vi "RT_Control_Adrian_AllIncluded_NoAngles.vi"(10 "rt fifo":refnum<k33>, 11 "Parameters":T1) -> (0 "error out":errorcluster, 2 "Delayed Cycles":dbl)   [LabVIEW 2021]
uses:
  parametersRT.ctl
  <vilib>/DAQmx/write.llb/DAQmx Write (Analog 1D DBL NChan 1Samp).vi
  <vilib>/DAQmx/read.llb/DAQmx Read (Analog 1D DBL NChan 1Samp).vi
  <vilib>/DAQmx/configure/timing.llb/DAQmx Timing (Sample Clock).vi
  <vilib>/DAQmx/miscellaneous.llb/DAQmx Fill In Error Info.vi
  <resource>/objmgr/daqmx.rc
panel:
  out "error out 7":errorcluster
  out "error out 6":errorcluster
  out "error out 5":errorcluster
  out "error out 4":errorcluster
  out "error out 2":errorcluster
  out "FB Raw Readings":dbl[][](array[numeric])
  in  "Stop Loop":bool
  in  "System Information":enum32{"RT System"}(tab)
  in  "source":tag
  in  "source 2":tag
  in  "RT Data Monitoring":enum32{"Forces", "Angles", "Power", "Pressure"}(tab)
  out "Bias Voltages":dbl[][](array[numeric])=[[-0.0710179470114859, -0.17463349299050945, -0.11016159714741332, 0.026018829634351103, 0.12897648926553976, 0.08259620236774425]]
  out "Bias Vector":dbl[](array[numeric])=[-0.0710179470114859, -0.17463349299050945, -0.11016159714741332, 0.026018829634351103, 0.12897648926553976, 0.08259620236774425]
  in  "Bias":bool
  in  "Unbias":bool
  # "Important! Set angle offset before reading angles"
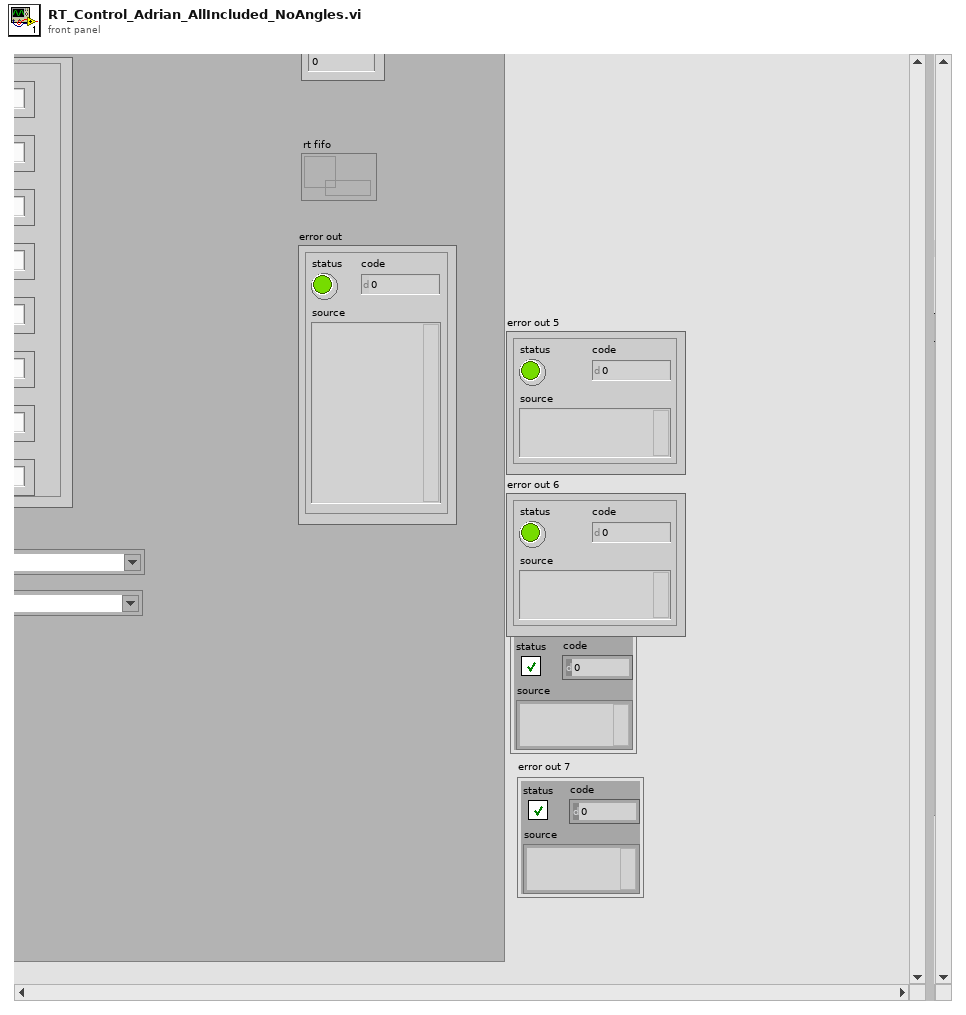
[diagram p1: front panel]
types:
  T1 = typedef "parametersRT.ctl" = cluster{"N_Signals_FIFO":u32, "Input Rate (Hz)":dbl, "Acq Time (s)":dbl, "NumOfWarmupIters":u32, "Size fifo":u32, "Period NCL (ms)":i64, "Timeout fifo Read":i32, "Size Sent Array":i32}
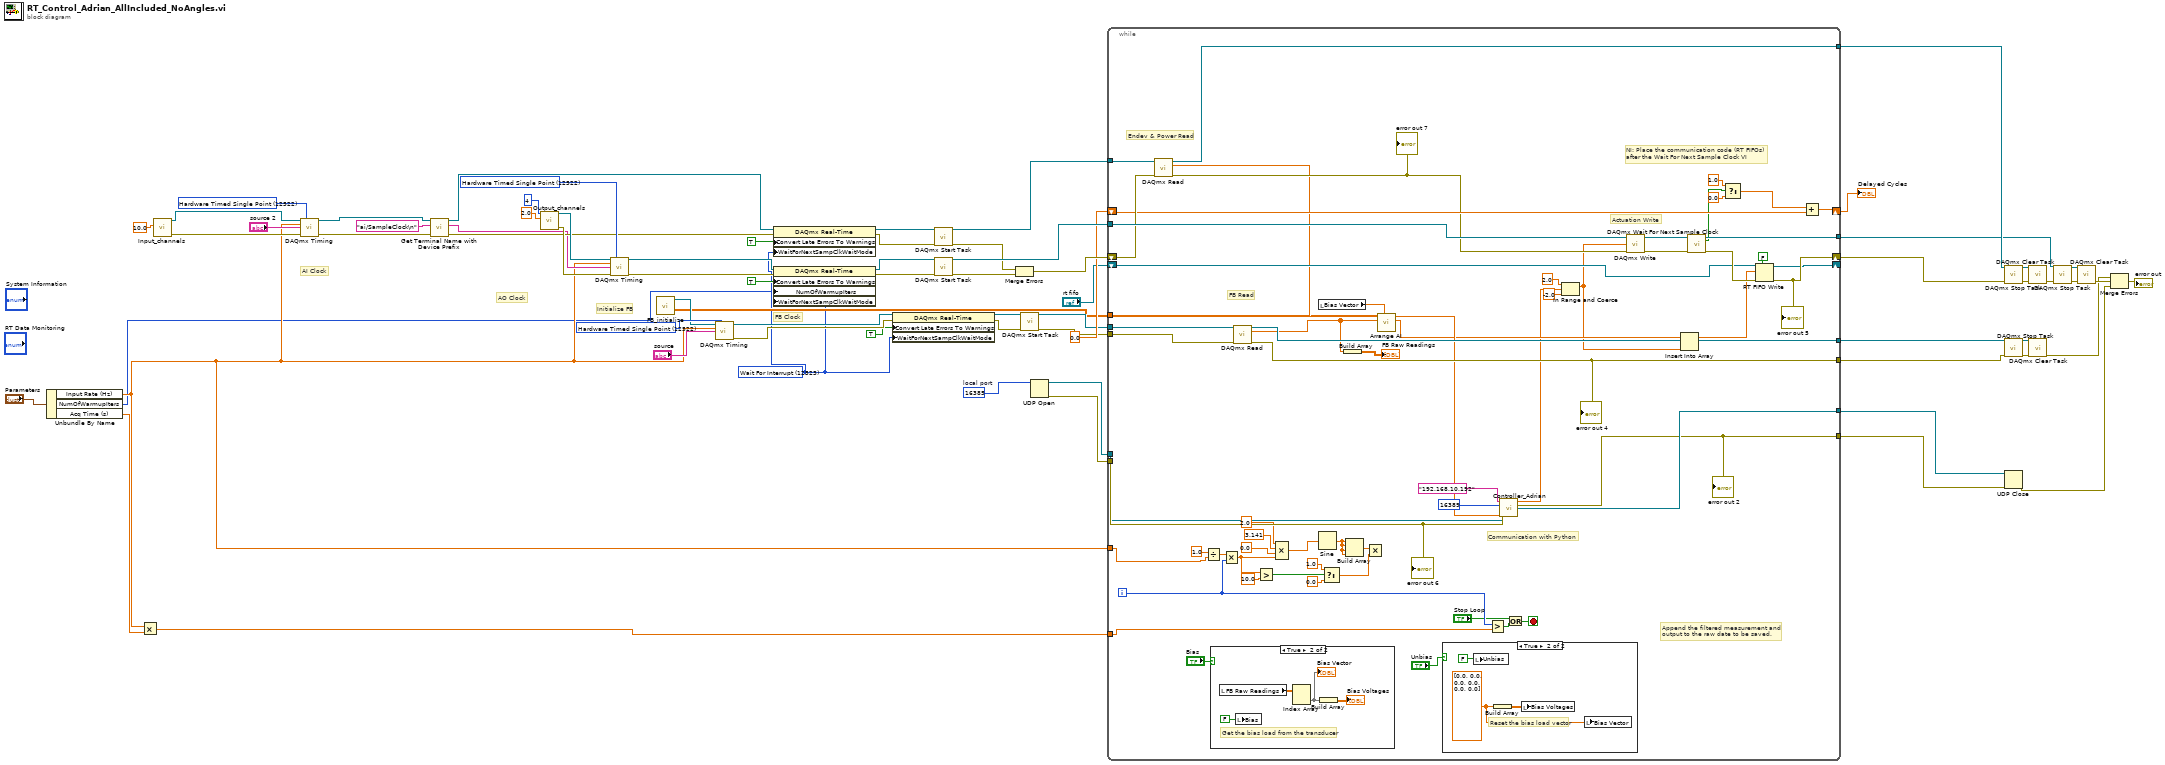
[diagram p0: block diagram]
diagram:
  w2 = 12523 items=["Wait For Interrupt"=12523, "Poll"=12524, "Yield"=12525] ("WaitForNextSampClkWaitMode")
  w34 = 12522 items=["Finite Samples"=10178, "Continuous Samples"=10123, "Hardware Timed Single Point"=12522] ("sample mode")
  w44 = u16 16385  # local port
  w51 = 12522 items=["Finite Samples"=10178, "Continuous Samples"=10123, "Hardware Timed Single Point"=12522] ("sample mode")
  w69 = 12522 items=["Finite Samples"=10178, "Continuous Samples"=10123, "Hardware Timed Single Point"=12522] ("sample mode")
  # "Initialize FB"
  # "AO Clock"
  # "AI Clock"
  # "FB Clock"
  n1 = Unbundle By Name("Parameters") -> ("Input Rate (Hz)"=w3:dbl, "NumOfWarmupIters"=w1:u32, "Acq Time (s)"=w64:dbl)
  n2 = Multiply(x=w3, y=w64) -> (x*y=w39:dbl)
  n3 = call "Input_channels.vi"("Range"=10.0) -> ("error out"=w53:errorcluster, "Refnum out"=w52:refnum<k21>)  [unwired: 9 in]
  n4 = call-poly <vilib>:"DAQmx Timing.vi"("task/channels in"=w52, "sample mode"=w51, "rate"=w3, "source"="source 2", "error in"=w53) -> ("task out"=w23:refnum<k21>, "error out"=w21:errorcluster)  [unwired: 9 in]
  n5 = call "Get Terminal Name with Device Prefix.vi"("error in (no error)"=w21, "Local Terminal Name"="ai/SampleClock\n", "task/channels in"=w23) -> ("error out"=w20:errorcluster, "Terminal Name with Device Prefix"=w19:tag, "task out"=w22:refnum<k21>)  [unwired: 6 in]
  n6 = call "Output_channels.vi"("Range"=2.0 ("Maximum Value"), "nchan"=4) -> ("error out"=w61:errorcluster, "Refnum out"=w60:refnum<k21>)  [unwired: 8 in]
  n7 = call-poly <vilib>:"DAQmx Timing.vi"("task/channels in"=w60, "sample mode"=w69, "rate"=w3, "source"=w19, "error in"=w61) -> ("task out"=w68:refnum<k21>, "error out"=w67:errorcluster)  [unwired: 9 in]
  n8 = call "FB_initialize.vi"() -> ("Transformed Calibration Matrix"=w27:dbl[][], "FB out"=w30:refnum<k21>)  [unwired: 9 in, 1 out]
  n9 = call-poly <vilib>:"DAQmx Timing.vi"("task/channels in"=w30, "sample mode"=w34, "rate"=w3, "source"="source") -> ("task out"=w36:refnum<k21>, "error out"=w35:errorcluster)  [unwired: 10 in]
  n10 = property class="DAQmx Real-Time"(reference=w22, error in=w20, "Convert Late Errors To Warnings"=TRUE, "WaitForNextSampClkWaitMode"=w2) -> (reference out=w48:refnum<k21>, error out=w47:errorcluster)
  n11 = property class="DAQmx Real-Time"(reference=w68, error in=w67, "Convert Late Errors To Warnings"=TRUE, "NumOfWarmupIters"=w1, "WaitForNextSampClkWaitMode"=w2) -> (reference out=w65:refnum<k21>, error out=w55:errorcluster)
  n12 = property class="DAQmx Real-Time"(reference=w36, error in=w35, "Convert Late Errors To Warnings"=TRUE ("ConvLateErrorsToWarnings"), "WaitForNextSampClkWaitMode"=w2) -> (reference out=w31:refnum<k21>, error out=w32:errorcluster)
  n13 = call <vilib>:"DAQmx Start Task.vi"("task/channels in"=w48, "error in"=w47) -> ("task out"=w63:refnum<k21>, "error out"=w46:errorcluster)  [unwired: 12 in]
  n14 = call <vilib>:"DAQmx Start Task.vi"("task/channels in"=w65, "error in"=w55) -> ("task out"=w62:refnum<k21>, "error out"=w54:errorcluster)  [unwired: 12 in]
  n15 = Merge Errors(w46, w54) -> (w45:errorcluster)
  n16 = call <vilib>:"DAQmx Start Task.vi"("task/channels in"=w31, "error in"=w32) -> ("task out"=w29:refnum<k21>, "error out"=w28:errorcluster)  [unwired: 12 in]
  n17 = UDP Open(11:w44) -> (port=w42:refnum<k16>, 0:w43:errorcluster)  [unwired: 4 in, 1 out]
  n18 = while {
    shift-right: [w105] -> w12
    shift-left: w45 -> [w125]
    shift-right: [w130] -> w70
    shift-left: 0.0 ("f") -> [w117]
    tunnel: w39 -> [w129]
    tunnel: w62 -> [w128]
    tunnel: [w126] -> w11
    tunnel: w63 -> [w127]
    tunnel: [w108] -> w7
    tunnel: w43 -> [w122]
    tunnel: w42 -> [w121]
    tunnel: [w120] -> w41
    tunnel: w29 -> [w116]
    tunnel: w28 -> [w115]
    tunnel: w27 -> [w78]
    tunnel: [w112] -> w17
    tunnel: [w111] -> w15
    shift-right: [w103] -> _
    shift-left: "rt fifo" -> [w102]
    tunnel: [w85] -> w4
    tunnel: w3 -> [w84]
    i -> [w96]
    stop <- w81 stop-if-true
    # "NI: Place the communication code (RT FIFOs) \nafter the Wait For Next Sample Clock VI"
    # "Communication with Python"
    # "Actuation Write"
    # "Endev & Power Read"
    # "FB Read"
    # "Append the filtered measurement and \noutput to the raw date to be saved."
    n19 = call-poly <vilib>:"DAQmx Read.vi"("task/channels in"=w127, "error in"=w125) -> ("task out"=w126:refnum<k21>, "data"=w80:dbl[], "error out"=w100:errorcluster)  [unwired: 11 in]
    "error out 7" <- w100
    n20 = Divide(x=1.0, y=w84) -> (x/y=w94:dbl)
    n21 = case shown="True" "Bias" {
      frame False {
      }
      frame True {
        # "Get the bias load from the transducer"
        n22 = local read "FB Raw Readings"() -> (w140:dbl[][])
        n23 = local write "Bias"(FALSE) -> ()
        n24 = Index Array(array=w140) -> (element=w137:dbl[])  [unwired: 2 in]
        "Bias Vector" <- w137
        n25 = Build Array(w137) -> (→"Bias Voltages":dbl[][])
      }
    }
    n26 = Multiply(x=w94, y=w96) -> (x*y=w90:dbl)
    n27 = call-poly <vilib>:"DAQmx Read.vi"("task/channels in"=w116, "error in"=w115) -> ("task out"=w112:refnum<k21>, "data"=w75:dbl[], "error out"=w111:errorcluster)  [unwired: 11 in]
    "error out 4" <- w111
    n28 = Greater?(x=w90, y=10.0) -> (0:w86:bool)
    n29 = Compound Arithmetic op=MULTIPLY(2.0 ("value"), 3.141 ("value"), 0.0 ("value"), w90) -> (w93:dbl)
    n30 = local read "Bias Vector"() -> (w79:dbl[])
    n31 = Sine(x=w93) -> (sin(x)=w92:dbl)
    n32 = Select(t=1.0, s=w86, f=0.0) -> (s? t:f=w76:dbl)
    n33 = Build Array(w75) -> (→"FB Raw Readings":dbl[][])
    n34 = Build Array(w92, w92, w92, w92) -> (w91:dbl[])
    n35 = Multiply(x=w91, y=w76) -> ()  [unwired: 1 out]
    n36 = call "Arrange AI.vi"("Transformed Calibration Matrix"=w78, "Bias Vector"=w79, "FB data"=w75, "EDV + Voltage data"=w80) -> ("FIFO Data (7EDV+3Force+4Power+4Voltage)"=w73:dbl[], "UDP Data (7EDV+3Force+4Power)"=w77:dbl[])  [unwired: 6 in]
    n37 = case shown="True" "Unbias" {
      frame False {
      }
      frame True {
        w135 = dbl[] [0.0, 0.0, 0.0, 0.0, 0.0, 0.0]
        # "Reset the bias load vector"
        n38 = local write "Unbias"(FALSE) -> ()
        n39 = Build Array(w135) -> (w134:dbl[][])
        n40 = local write "Bias Voltages"(w134) -> ()
        n41 = local write "Bias Vector"(w135) -> ()
      }
    }
    n42 = Greater?(x=w96, y=w129) -> (0:w82:bool)
    n43 = call "Controller_Adrian.vi"("name 2"="192.168.10.192", "port or service name"=u16 16389, "connection ID"=w121, "error in (no error)"=w122, "x"=w77) -> ("*(type *) &x"=w71:dbl[], "error out"=w85:errorcluster, "connection ID out"=w120:refnum<k16>)  [unwired: 8 in]
    "error out 2" <- w85
    n44 = Or(x="Stop Loop", y=w82) -> (x .or. y?=w81:bool)
    n45 = In Range and Coerce(upper limit=2.0, x=w71, lower limit=-2.0) -> (coerced(x)=w72:dbl[])  [unwired: 1 out]
    n46 = call-poly <vilib>:"DAQmx Write.vi"("task/channels in"=w128, "data"=w72, "error in"=w100) -> ("task out"=w109:refnum<k21>, "error out"=w110:errorcluster)  [unwired: 10 in, 1 out]
    n47 = Insert Into Array(array=w73, new element=w72) -> (w101:dbl[])  [unwired: 1 in]
    n48 = call <vilib>:"DAQmx Wait For Next Sample Clock.vi"("task/channels in"=w109, "error in"=w110) -> ("task out"=w108:refnum<k21>, "is late?"=w107:bool, "error out"=w104:errorcluster)  [unwired: 11 in]
    n49 = Select(t=1.0, s=w107, f=0.0) -> (s? t:f=w131:dbl)
    n50 = RT FIFO Write(0:w102, 1:w101, 3:w104, 5:FALSE ("overwrite on timeout (T)")) -> (8:w103:refnum<k33>, 11:w105:errorcluster)  [unwired: 1 in, 2 out]
    "error out 5" <- w105
    n51 = Add(x=w131, y=w117) -> (x+y=w130:dbl)
    "error out 6" <- w122
  }
  "Delayed Cycles" <- w70
  n52 = call <vilib>:"DAQmx Stop Task.vi"("task/channels in"=w11, "error in"=w12) -> ("task out"=w10:refnum<k21>, "error out"=w13:errorcluster)  [unwired: 12 in]
  n53 = call <vilib>:"DAQmx Stop Task.vi"("task/channels in"=w17, "error in"=w15) -> ("task out"=w16:refnum<k21>, "error out"=w14:errorcluster)  [unwired: 12 in]
  n54 = UDP Close(connection ID=w41, 8:w4) -> (error out=w40:errorcluster)  [unwired: 1 out]
  n55 = call <vilib>:"DAQmx Clear Task.vi"("task in"=w10, "error in"=w13) -> ("error out"=w9:errorcluster)  [unwired: 13 in]
  n56 = call <vilib>:"DAQmx Clear Task.vi"("task in"=w16, "error in"=w14) -> ("error out"=w26:errorcluster)  [unwired: 13 in]
  n57 = call <vilib>:"DAQmx Stop Task.vi"("task/channels in"=w7, "error in"=w9) -> ("task out"=w6:refnum<k21>, "error out"=w8:errorcluster)  [unwired: 12 in]
  n58 = call <vilib>:"DAQmx Clear Task.vi"("task in"=w6, "error in"=w8) -> ("error out"=w57:errorcluster)  [unwired: 13 in]
  n59 = Merge Errors(w26, w57, w40) -> (→"error out":errorcluster)
